vi "General_Test.vi"(8 "error in":errorcluster, 11 "Daten":T2={"Report.lvclass"=refnum, "Norm"="", "last State"=enum."Initialize", "Norm ID"=0, "parameter"=[], "EMTestCWS500N.lvclass"=refnum, "CEG4500.lvclass"=refnum, "Tektronix RSA5106A.lvclass"=refnum, "erfolgreich"=FALSE, "log"="", "Kommentar"="", "Device Enum"=enum."emTestCWS500N", "Test Enum"=enum."HF-Felder", "debug"=FALSE}) -> (0 "error out":errorcluster, 1 "Log":string, 2 "Daten out":T2={"Report.lvclass"=refnum, "Norm"="", "last State"=enum."Initialize", "Norm ID"=0, "parameter"=[], "EMTestCWS500N.lvclass"=refnum, "CEG4500.lvclass"=refnum, "Tektronix RSA5106A.lvclass"=refnum, "erfolgreich"=FALSE, "log"="", "Kommentar"="", "Device Enum"=enum."emTestCWS500N", "Test Enum"=enum."HF-Felder", "debug"=FALSE})   [LabVIEW 2013, in "EMV-Test.lvlib"]
uses:
  lib/EMV-Test.lvlib
  classes/Tests/TestInterface/Tests.ctl
  classes/Devices/DeviceInterface/Devices.ctl
  Main/controls/Data.ctl
  classes/Datastructure/Report/Report.lvclass
  classes/Devices/emTestCWS500N/EMTestCWS500N.lvclass
  classes/Devices/CEG4500/CEG4500.lvclass
  classes/Devices/Tektronix RSA5106A/Tektronix RSA5106A.lvclass
  Main/controls/State.ctl
  Main/controls/generalTestStates.ctl
  Main/controls/TestData.ctl
  Main/controls/TestStates.ctl
  lib/button_states.ctl
  classes/Devices/DeviceInterface/DeviceInterface.lvclass
  classes/Tests/TestInterface/TestInterface.lvclass
panel:
  in  "save Test":bool
  out "Status":T1
  in  "Custom Button 2":bool
  in  "Custom Button 1":bool
  in  "Button Referenzen":refnum<vi>[](array[refnum])
  in  "Neustart":bool
  out "device":T4=enum."Tektronix RSA5106A"
  out "test":T5=enum."Störaussendung"
  out "Parameter table":string[][](table) caption="Parameter"
  out "VISA resource name":refnum<visa-resource-name>="COM5"
  in  "Kommentar":string
  in  "Pause":bool
  in  "aktueller Test":string
  in  "manuell":bool
  in  "test laden":bool
  in  "Start":bool
  in  "Beenden":bool
  out "start":dbl format="%_19f"
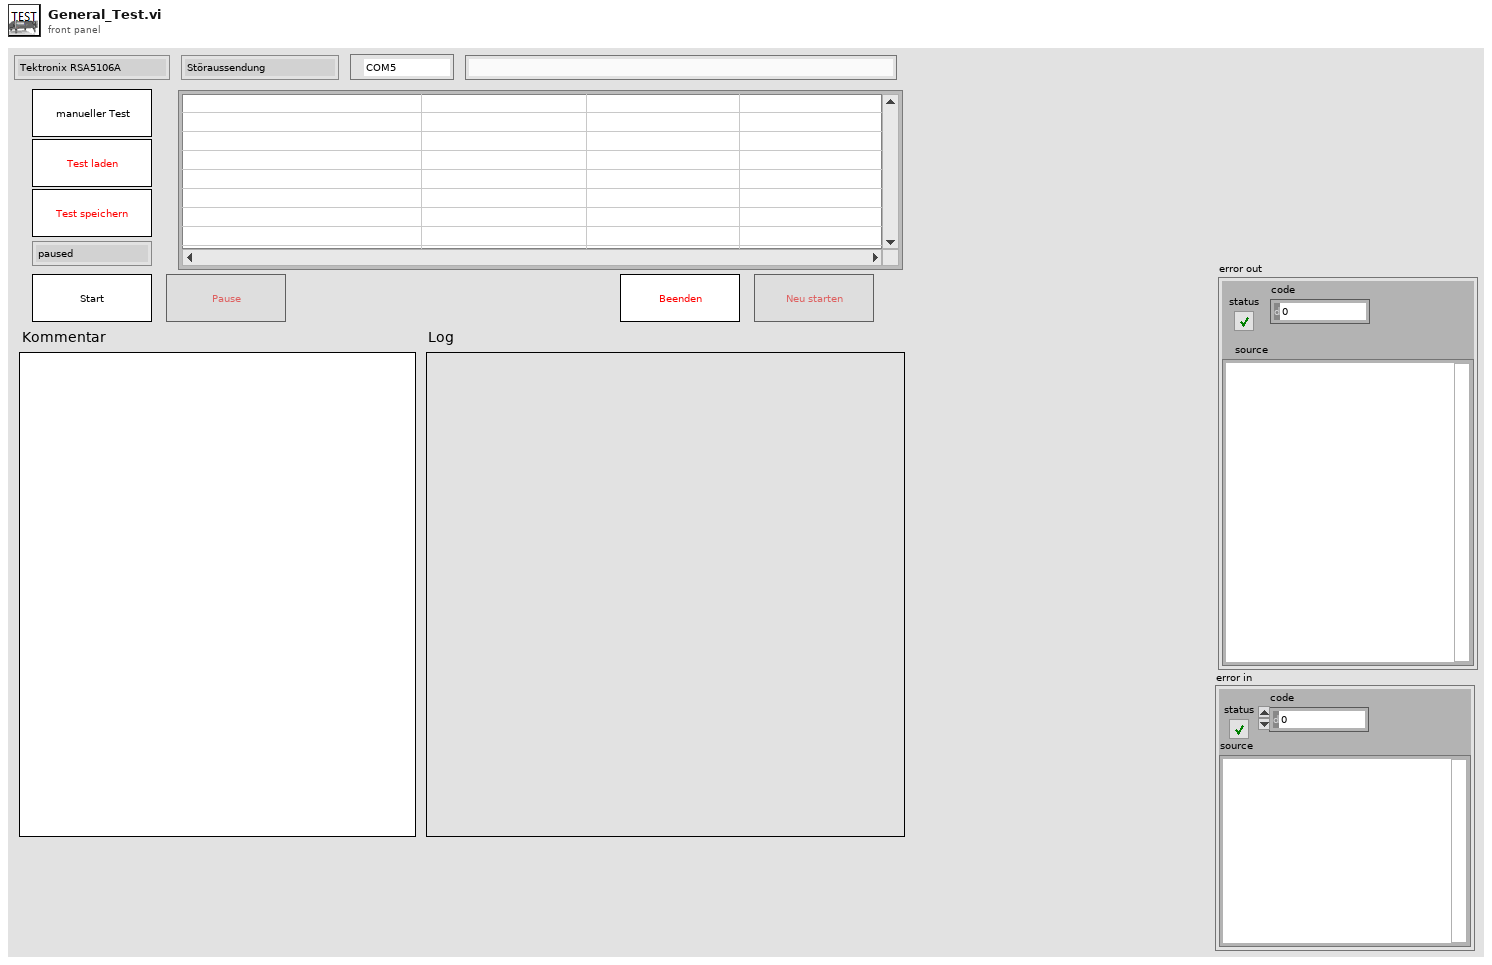
[diagram p1: front panel]
types:
  T1 = typedef "generalTestStates.ctl" = enum16{"paused", "starting", "waiting", "running", "finished"}
  T2 = typedef "Data.ctl" = cluster{"Report.lvclass":refnum<class "Report.lvclass">, "Norm":string, "last State":T3, "Norm ID":i32, "parameter":string[][], "EMTestCWS500N.lvclass":refnum<class "EMTestCWS500N.lvclass">, "CEG4500.lvclass":refnum<class "CEG4500.lvclass">, "Tektronix RSA5106A.lvclass":refnum<class "Tektronix RSA5106A.lvclass">, "erfolgreich":bool, "log":string, "Kommentar":string, "Device Enum":T4, "Test Enum":T5, "debug":bool}
  T3 = typedef "State.ctl" = enum16{"create Pdf", "load Report", "save Report", "do Test", "CDN Kalibrierung", "enter Report Parameters", "new Test", "Protokoll", "read Tree", "update Tree", "Fehler", "Initialize", "Wait for Event", "Exit"}
  T4 = typedef "Devices.ctl" = enum16{"unbekannt", "Tektronix RSA5106A", "emTestCWS500N", "CEG-4500"}
  T5 = typedef "Tests.ctl" = enum16{"unbekannt", "Störaussendung", "Burst", "ESD", "Surge", "Spannungseinbruch", "HF-Felder"}
  T6 = typedef "EMV-Test.lvlib/button_states.ctl" = enum16{"ende", "computing", "pause", "running", "start"}
  T7 = typedef "EMV-Test.lvlib/TestStates.ctl" = enum16{"event loop", "save Test", "Custom Action 1", "Custom Action 2", "pause", "vorgefertigter Test", "manueller Test", "respond to response", "error", "init", "start Test", "evaluate line", "wait for Response", "wait", "catch error", "close Connection", "end"}
  T8 = typedef "EMV-Test.lvlib/TestData.ctl" = cluster{"commandlist":string, "line":i32, "last response":string, "timeout":i32, "wait":u32, "erfolgreich":bool, "next state":T7, "Zustand":T1, "manual Test":bool}
  T9 = enum16{"open", "replace", "create", "open or create", "replace or create", "replace or create with confirmation"}
  T10 = enum16{"Left Button", "Center Button", "Right Button", "Window Close"}
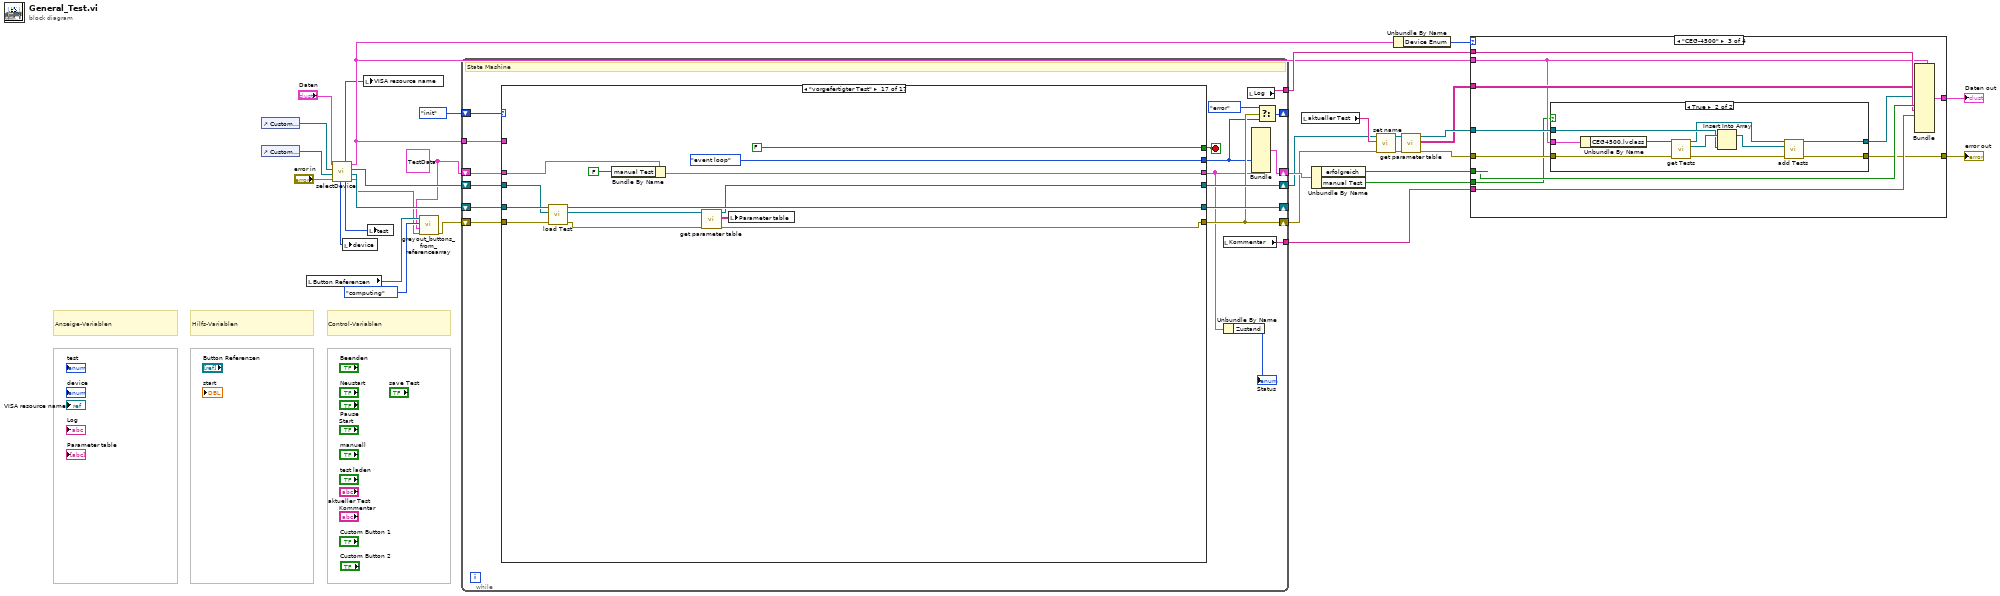
[diagram p0: block diagram]
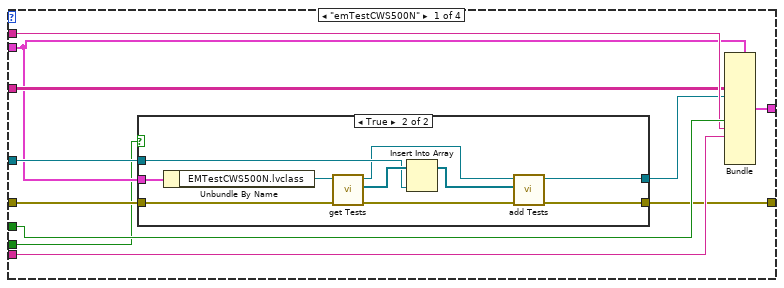
[diagram p2: hidden frame]
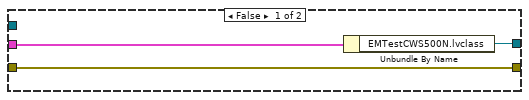
[diagram p3: hidden frame]
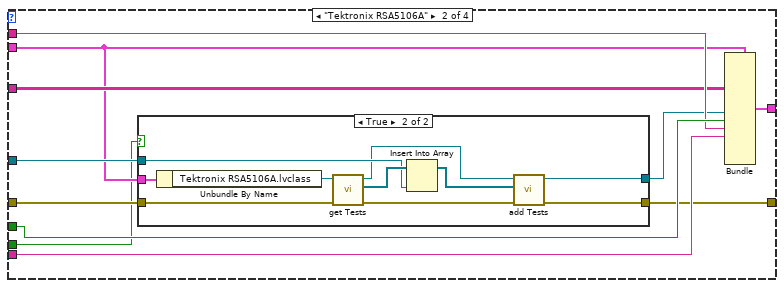
[diagram p4: hidden frame]
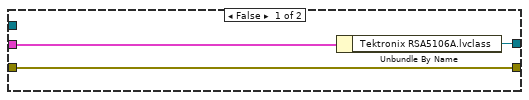
[diagram p5: hidden frame]
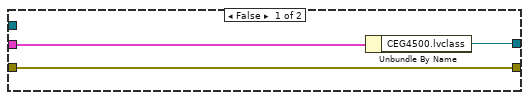
[diagram p6: hidden frame]
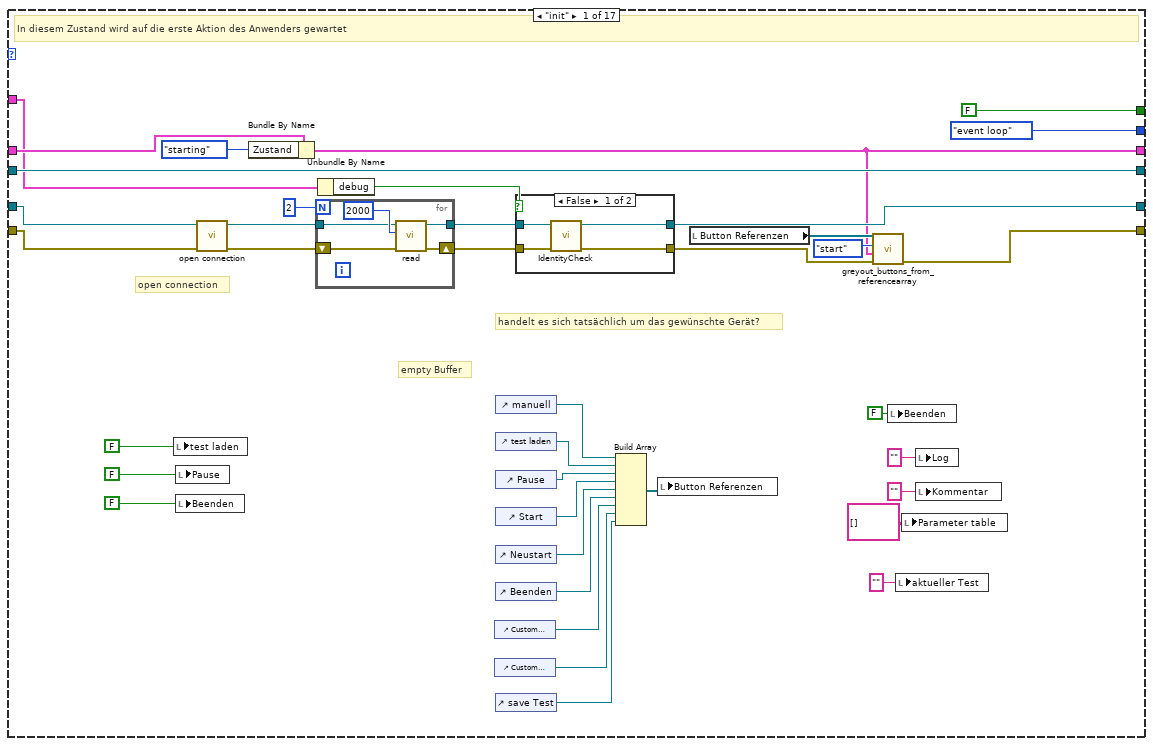
[diagram p8: hidden frame]
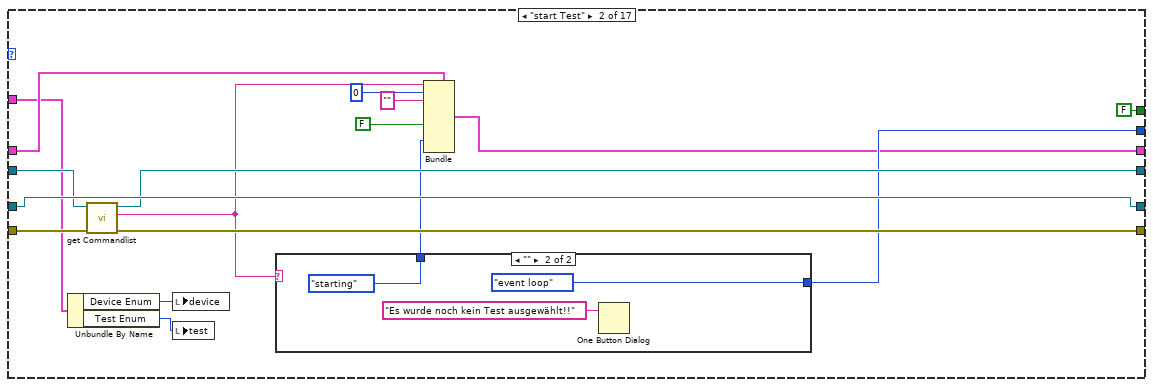
[diagram p10: hidden frame]
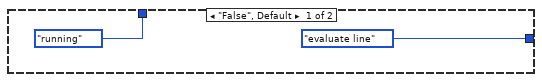
[diagram p11: hidden frame]
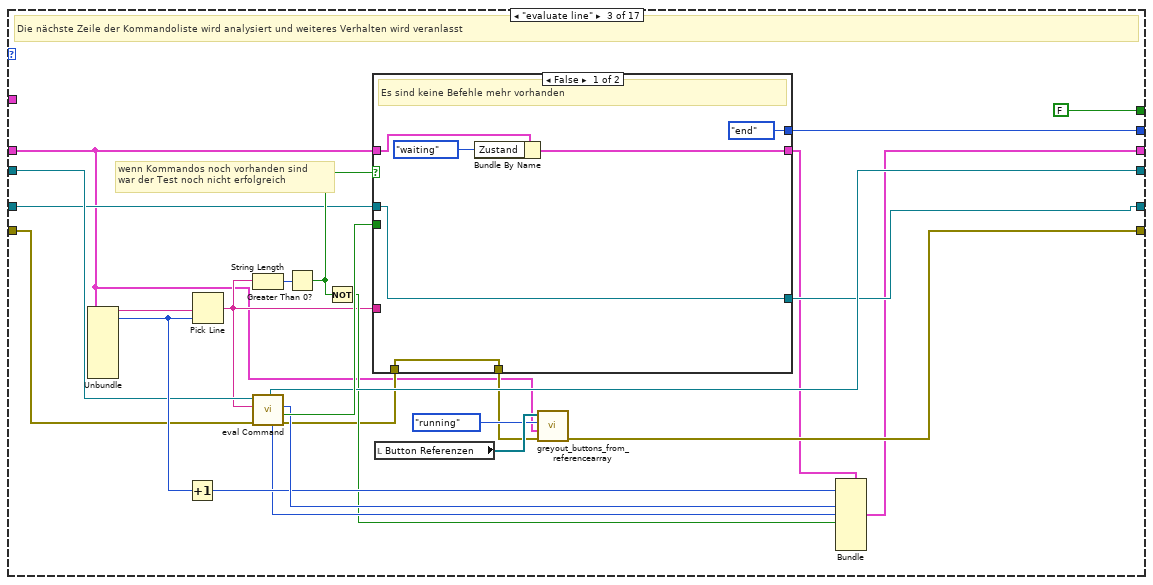
[diagram p12: hidden frame]
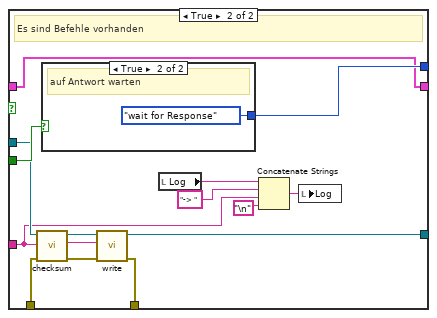
[diagram p13: hidden frame]
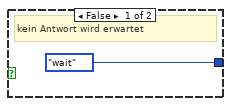
[diagram p14: hidden frame]
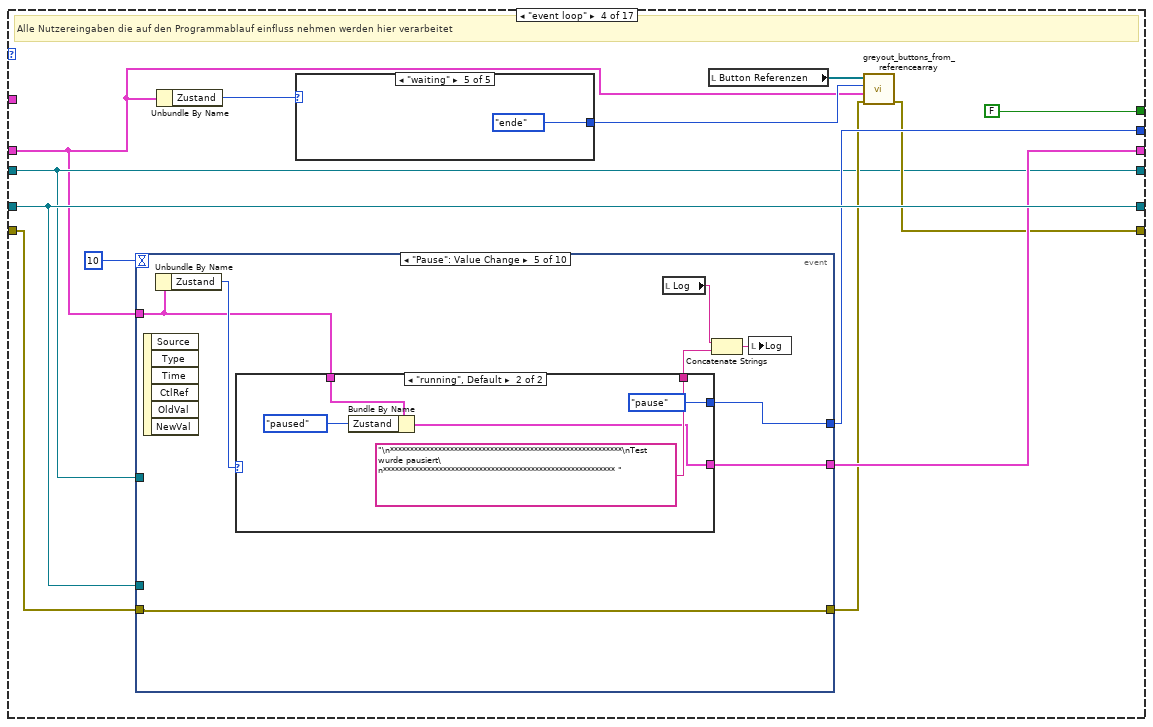
[diagram p15: hidden frame]
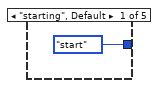
[diagram p16: hidden frame]
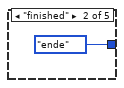
[diagram p17: hidden frame]
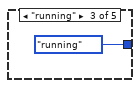
[diagram p18: hidden frame]
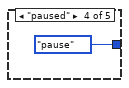
[diagram p19: hidden frame]
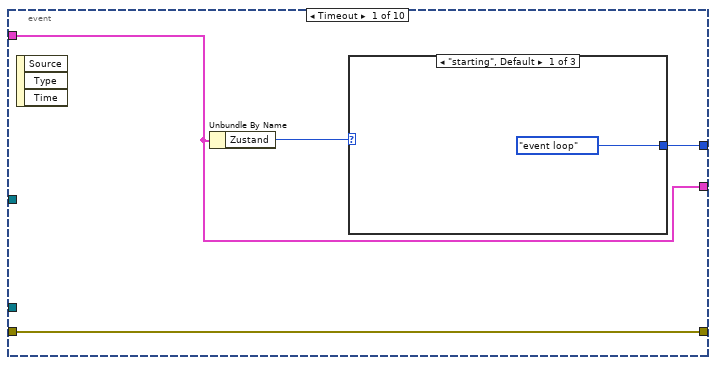
[diagram p20: hidden frame]
diagram:
  w3 = T8 {"commandlist"="", "line"=0, "last response"="", "timeout"=0, "wait"=0, "erfolgreich"=FALSE, "next state"=enum."event loop", "Zustand"=enum."starting", "manual Test"=FALSE}
  # "Hilfs-Variablen"
  # "Anzeige-Variablen"
  # "Control-Variablen"
  n1 = control-ref of="Custom Button 2"() -> (w24:refnum<vi>)
  n2 = control-ref of="Custom Button 1"() -> (w23:refnum<vi>)
  n3 = local read "Button Referenzen"() -> (w4:refnum<vi>[])
  n4 = call "selectDevice.vi"("error in (no error)"="error in", "Custom Button 1"=w23, "Custom Button 2"=w24, "Daten in"="Daten") -> ("error out"=w2:errorcluster, "DeviceInterface out"=w21:refnum<class "DeviceInterface.lvclass">, "Burst.lvclass"=w20:refnum<class "TestInterface.lvclass">, "Daten out"=w17:T2, "Test Enum"=w7:T5, "VISA resource name"=w6:refnum<visa-resource-name>, "Device Enum"=w8:T4)  [unwired: 1 in]
  n5 = local write "device"(w8) -> ()
  n6 = local write "VISA resource name"(w6) -> ()
  n7 = local write "test"(w7) -> ()
  n8 = call "greyout_buttons_from_referencearray.vi"("error in (no error)"=w2, 9:w3, "Enum"=button_states."computing", "Array"=w4) -> ("error out"=w1:errorcluster)  [unwired: 7 in]
  n9 = while {
    shift-right: [w41] -> _
    shift-left: TestStates."init" ("Enum") -> [w46]
    shift-right: [w39] -> w25
    shift-left: w1 -> [w44]
    shift-right: [w37] -> w32
    shift-left: w3 -> [w50]
    shift-right: [w43] -> _
    shift-left: w21 -> [w48]
    shift-right: [w47] -> w26
    shift-left: w20 -> [w45]
    tunnel: [w42] -> w29
    tunnel: [w36] -> w28
    tunnel: w17 -> [w33]
    stop <- w49 stop-if-true
    # "State Mashine"
    n10 = case shown="\"vorgefertigter Test\"" w46 {
      tunnel: w44 -> [w76 w111 w136 w179 w278 w310 w367 w390 w398 _ w441 w460 w469 w514 w537 w548 w565]
      tunnel: [w83 w108 w131 w174 w280 w320 w354 w390 w402 errorcluster {"status"=FALSE, "code"=0, "source"=""} ("error out") w424 w463 errorcluster {"status"=FALSE, "code"=0, "source"=""} ("error out") w507 w521 w548 w556] -> w39
      tunnel: [TestStates."event loop" ("Enum") w106 w125 w178 w272 w313 TestStates."catch error" ("Enum") TestStates."event loop" ("Enum") w401 TestStates."end" ("Enum") TestStates."event loop" ("Enum") w458 w474 w506 TestStates."event loop" ("Enum") TestStates."event loop" ("Enum") TestStates."event loop" ("Enum")] -> w38
      tunnel: w50 -> [w79 w115 w122 w170 w273 w315 w362 w388 w400 w415 w455 w457 w473 w508 w529 w551 w560]
      tunnel: [w66 w105 w123 w177 w274 w317 w363 w388 w400 w415 w455 w457 w472 w505 w527 w551 w558] -> w35
      tunnel: [FALSE FALSE FALSE FALSE FALSE FALSE FALSE FALSE FALSE TRUE FALSE FALSE FALSE FALSE FALSE FALSE FALSE] -> w49
      tunnel: w48 -> [w77 w112 w129 w180 w279 w316 w356 w392 w399 w419 w456 w464 w485 w511 w538 w549 w566]
      tunnel: w45 -> [w86 w110 w137 w171 w276 w311 w360 w393 w404 w420 w423 w461 w470 w513 w533 w550 w562]
      tunnel: [w86 w109 w141 w171 w275 w318 w360 w393 w404 w420 w423 w461 w470 w510 w523 w550 w555] -> w47
      tunnel: [w87 w112 w128 w180 w277 w319 w356 w392 w403 w419 w456 w464 w485 w511 w538 w549 w563] -> w43
      tunnel: w33 -> [w70 w100 _ _ w270 w307 _ _ _ w414 _ _ _ _ _ _ _]
      frame "init" {
        # "open connection"
        # "empty Buffer"
        # "handelt es sich tatsächlich um das gewünschte Gerät?"
        # "In diesem Zustand wird auf die erste Aktion des Anwenders gewartet"
        n11 = local write "test laden"(FALSE ("Beenden")) -> ()
        n12 = local write "Pause"(FALSE ("Beenden")) -> ()
        n13 = local write "Beenden"(FALSE ("Beenden")) -> ()
        n14 = call-dynamic "open connection.vi"("error in (no error)"=w76, "DeviceInterface Eingang"=w77) -> ("error out"=w73:errorcluster, "DeviceInterface Ausgang"=w74:refnum<class "DeviceInterface.lvclass">)  [unwired: 8 in]
        n15 = Bundle By Name(cluster=w79, "Zustand"=generalTestStates."starting") -> (w66:T8)
        n16 = for {
          N: 2 -> [_]
          tunnel: w74 -> [w90]
          shift-right: [w92] -> w71
          shift-left: w73 -> [w93]
          tunnel: [w89] -> w72
          n17 = call-dynamic "read.vi"("error in (no error)"=w93, "timeout (ms)"=2000, "DeviceInterface in"=w90) -> ("error out"=w92:errorcluster, "DeviceInterface out"=w89:refnum<class "DeviceInterface.lvclass">)  [unwired: 6 in, 1 out]
        }
        n18 = Unbundle By Name(w70) -> ("debug"=w85:bool)
        n19 = control-ref of="Custom Button 1"() -> (w62:refnum<vi>)
        n20 = control-ref of="Custom Button 2"() -> (w63:refnum<vi>)
        n21 = control-ref of="manuell"() -> (w59:refnum<vi>)
        n22 = control-ref of="test laden"() -> (w58:refnum<vi>)
        n23 = control-ref of="Pause"() -> (w57:refnum<vi>)
        n24 = control-ref of="Start"() -> (w56:refnum<vi>)
        n25 = control-ref of="Neustart"() -> (w55:refnum<vi>)
        n26 = control-ref of="Beenden"() -> (w61:refnum<vi>)
        n27 = control-ref of="save Test"() -> (w51:refnum<vi>)
        n28 = case shown="False" w85 {
          tunnel: w72 -> [w97 w99]
          tunnel: [w96 w99] -> w87
          tunnel: [w95 w98] -> w84
          tunnel: w71 -> [w94 w98]
          frame False {
            n29 = call-dynamic "IdentityCheck.vi"("error in (no error)"=w94, "DeviceInterface in"=w97) -> ("error out"=w95:errorcluster, "DeviceInterface out"=w96:refnum<class "DeviceInterface.lvclass">)  [unwired: 8 in]
          }
          frame True {
          }
        }
        n30 = Build Array(w59, w58, w57, w56, w55, w61, w62, w63, w51) -> (w60:refnum<vi>[])
        n31 = local write "Button Referenzen"(w60) -> ()
        n32 = local read "Button Referenzen"() -> (w82:refnum<vi>[])
        n33 = call "greyout_buttons_from_referencearray.vi"("error in (no error)"=w84, 9:w66, "Enum"=button_states."start", "Array"=w82) -> ("error out"=w83:errorcluster)  [unwired: 7 in]
        n34 = local write "Beenden"(FALSE ("Beenden")) -> ()
        n35 = local write "aktueller Test"("" ("Kommentar")) -> ()
        n36 = local write "Parameter table"(string[][] [] ("Parameter")) -> ()
        n37 = local write "Log"("" ("Log")) -> ()
        n38 = local write "Kommentar"("" ("Kommentar")) -> ()
      }
      frame "start Test" {
        n39 = Unbundle By Name(w100) -> ("Device Enum"=w101:T4, "Test Enum"=w102:T5)
        n40 = call-dynamic "get Commandlist.vi"("error in (no error)"=w111, "TestInterface (Eingang)"=w110) -> ("error out"=w108:errorcluster, "Commandlist"=w104:string, "TestInterface (Ausgang)"=w109:refnum<class "TestInterface.lvclass">)  [unwired: 7 in]
        n41 = local write "device"(w101) -> ()
        n42 = local write "test"(w102) -> ()
        n43 = case shown="\"\"" w104 {
          tunnel: [TestStates."evaluate line" ("Enum") TestStates."event loop" ("Enum")] -> w106
          tunnel: [generalTestStates."running" ("Zustand") generalTestStates."starting" ("Zustand")] -> w103
          frame "False", Default {
          }
          frame "" {
            n44 = One Button Dialog(message="Es wurde noch kein Test ausgewählt!!" ("Nachricht")) -> ()  [unwired: 1 in, 1 out]
          }
        }
        n45 = Bundle(cluster=w115, "commandlist"=w104, "line"=0, "last response"="", "erfolgreich"=FALSE, "Zustand"=w103) -> (w105:T8)  [unwired: 4 in]
      }
      frame "evaluate line" {
        # "wenn Kommandos noch vorhanden sind\nwar der Test noch nicht erfolgreich"
        # "Die nächste Zeile der Kommandoliste wird analysiert und weiteres Verhalten wird veranlasst"
        n46 = Unbundle(w122) -> ("commandlist"=w139:string, "line"=w144:i32)  [unwired: 7 out]
        n47 = Increment(x=w144) -> (x+1=w140:i32)
        n48 = Pick Line(multi-line string=w139, line index=w144) -> (output string=w130:string)  [unwired: 1 in]
        n49 = String Length(string=w130) -> (length=w146:i32)
        n50 = call "eval Command.vi"("error in (no error)"=w136, "Commandline"=w130, "TestInterface.lvclass"=w137) -> ("error out"=w127:errorcluster, "isQuerry"=w145:bool, "timeout(ms)"=w142:i32, "TestInterface.lvclass 2"=w141:refnum<class "TestInterface.lvclass">, "wait"=w138:u32)  [unwired: 4 in]
        n51 = Greater Than 0?(x=w146) -> (x > 0?=w134:bool)
        n52 = Not(x=w134) -> (.not. x?=w135:bool)
        n53 = case shown="False" w134 {
          tunnel: [TestStates."end" ("Enum") w166] -> w125
          tunnel: w145 -> [_ w167]
          tunnel: w130 -> [_ w154]
          tunnel: w129 -> [w150 w165]
          tunnel: w127 -> [w151 w164]
          tunnel: [w150 w160] -> w128
          tunnel: [w151 w159] -> w126
          tunnel: w122 -> [w149 w153]
          tunnel: [w147 w153] -> w124
          frame False {
            # "Es sind keine Befehle mehr vorhanden"
            n54 = Bundle By Name(cluster=w149, "Zustand"=generalTestStates."waiting") -> (w147:T8)
          }
          frame True {
            # "Es sind Befehle vorhanden"
            n55 = call-dynamic "checksum.vi"("error in (no error)"=w164, "input"=w154, "DeviceInterface in"=w165) -> ("error out"=w161:errorcluster, "output"=w162:string, "DeviceInterface out"=w163:refnum<class "DeviceInterface.lvclass">)  [unwired: 6 in]
            n56 = case shown="True" w167 {
              tunnel: [TestStates."wait" ("Enum") TestStates."wait for Response" ("Enum")] -> w166
              frame False {
                # "kein Antwort wird erwartet"
              }
              frame True {
                # "auf Antwort warten"
              }
            }
            n57 = call-dynamic "write.vi"("error in (no error)"=w161, "String to send"=w162, "DeviceInterface in"=w163) -> ("error out"=w159:errorcluster, "DeviceInterface out"=w160:refnum<class "DeviceInterface.lvclass">)  [unwired: 7 in]
            n58 = local read "Log"() -> (w158:string)
            n59 = Concatenate Strings(w158, "-> " ("string"), w154, "\n") -> (w156:string)
            n60 = local write "Log"(w156) -> ()
          }
        }
        n61 = local read "Button Referenzen"() -> (w133:refnum<vi>[])
        n62 = call "greyout_buttons_from_referencearray.vi"("error in (no error)"=w126, 9:w122, "Enum"=button_states."running", "Array"=w133) -> ("error out"=w131:errorcluster)  [unwired: 7 in]
        n63 = Bundle(cluster=w124, "line"=w140, "timeout"=w142, "wait"=w138, "erfolgreich"=w135) -> (w123:T8)  [unwired: 5 in]
      }
      frame "event loop" {
        # "Alle Nutzereingaben die auf den Programmablauf einfluss nehmen werden hier verarbeitet"
        n64 = event shown="[4] \"Pause\": Value Change" {
          selector: _ -> [_ _ _ _ _ _ _ _ _ _]
          dyn-events: _ -> [_ _ _ _ _ _ _ _ _ _]
          timeout: 10 -> [_ _ _ _ _ _ _ _ _ _]
          tunnel: [w190 w198 w199 w210 w218 w234 w246 w259 w265 w268] -> w175
          tunnel: w179 -> [w190 w198 w209 w210 w218 w234 w247 w259 w265 w268]
          tunnel: w180 -> [_ _ w208 _ _ _ _ _ _ _]
          tunnel: [w191 TestStates."manueller Test" ("Enum") TestStates."init" ("Enum") TestStates."save Test" ("Enum") w213 TestStates."end" ("Enum") TestStates."start Test" ("Enum") TestStates."vorgefertigter Test" ("Enum") TestStates."Custom Action 1" ("Enum") TestStates."Custom Action 2" ("Enum")] -> w178
          tunnel: w170 -> [w188 w196 w202 w211 w215 w233 w249 w260 w263 w267]
          tunnel: [w188 w196 w200 w211 w214 w231 w249 w260 w263 w267] -> w177
          tunnel: w171 -> [_ _ _ _ _ _ w245 _ _ _]
          event Timeout {
            n65 = event-data() -> ()  [unwired: 1 in, 3 out]
            n66 = Unbundle By Name(w188) -> ("Zustand"=w189:T1)
            n67 = case shown="\"starting\", Default" w189 {
              tunnel: [TestStates."event loop" ("Enum") TestStates."pause" ("Enum") TestStates."evaluate line" ("Enum")] -> w191
              frame "starting", Default {
              }
              frame "paused" {
              }
              frame "running" {
              }
            }
          }
          event "manuell": Value Change {
            n68 = event-data() -> ()  [unwired: 1 in, 6 out]
            n69 = local write "manuell"(FALSE ("manuell")) -> ()
          }
          event "Neustart": Value Change {
            n70 = event-data() -> ()  [unwired: 1 in, 6 out]
            n71 = call-dynamic "close connection.vi"("error in (no error)"=w209, "DeviceInterface in"=w208) -> ("error out"=w199:errorcluster)  [unwired: 8 in, 1 out]
            n72 = Bundle By Name(cluster=w202, "Zustand"=generalTestStates."starting") -> (w200:T8)
            n73 = local write "Neustart"(FALSE ("Neustart")) -> ()
            n74 = local read "Log"() -> (w205:string)
            n75 = Concatenate Strings(w205, "\n**********************************************************\nTest wurde neugestartet\n********************************************************** " ("string")) -> (w204:string)
            n76 = local write "Log"(w204) -> ()
          }
          event "save Test": Value Change {
            n77 = event-data() -> ()  [unwired: 1 in, 6 out]
          }
          event "Pause": Value Change {
            n78 = event-data() -> ()  [unwired: 1 in, 6 out]
            n79 = Unbundle By Name(w215) -> ("Zustand"=w216:T1)
            n80 = case shown="\"running\", Default" w216 {
              tunnel: ["\n**********************************************************\nTest wurde wiederaufgenommen\n********************************************************** " ("string") "\n**********************************************************\nTest wurde pausiert\n********************************************************** " ("string")] -> w217
              tunnel: w215 -> [w224 w229]
              tunnel: [w222 w227] -> w214
              tunnel: [TestStates."event loop" ("Enum") TestStates."pause" ("Enum")] -> w213
              frame "paused" {
                n81 = Bundle By Name(cluster=w224, "Zustand"=generalTestStates."running") -> (w222:T8)
              }
              frame "running", Default {
                n82 = Bundle By Name(cluster=w229, "Zustand"=generalTestStates."paused") -> (w227:T8)
              }
            }
            n83 = local read "Log"() -> (w220:string)
            n84 = Concatenate Strings(w220, w217) -> (w219:string)
            n85 = local write "Log"(w219) -> ()
          }
          event "Beenden": Value Change {
            n86 = event-data() -> ()  [unwired: 1 in, 6 out]
            n87 = Unbundle By Name(w233) -> ("erfolgreich"=w235:bool)
            n88 = case shown="False" w235 {
              tunnel: ["\n**********************************************************\nTest wurde erfolgreich beendet\n**********************************************************" ("string") "\n**********************************************************\nTest wurde durch den Anwender beendet\n**********************************************************" ("string")] -> w237
              frame True {
              }
              frame False {
              }
            }
            n89 = Bundle By Name(cluster=w233, "Zustand"=generalTestStates."finished") -> (w231:T8)
            n90 = local read "Log"() -> (w239:string)
            n91 = Concatenate Strings(w239, w237) -> (w238:string)
            n92 = local write "Log"(w238) -> ()
          }
          event "Start": Value Change {
            w243 = "\"" ("string")
            n93 = event-data() -> ()  [unwired: 1 in, 6 out]
            n94 = call-dynamic "get name.vi"("error in (no error)"=w247, "TestInterface (Eingang)"=w245) -> ("error out"=w246:errorcluster, "name"=w244:string)  [unwired: 7 in, 1 out]
            n95 = local write "Start"(FALSE ("Start")) -> ()
            n96 = local read "Log"() -> (w255:string)
            n97 = Get Date/Time String(want seconds? (F)=TRUE) -> (date string=w251:string, time string=w250:string)  [unwired: 2 out]
            n98 = call <vilib>:"Space Constant.vi"() -> ("String"=w252:string)
            n99 = Concatenate Strings(w255, "\n**********************************************************\nTest gestartet " ("string"), w251, w252, w250, w243, w244, w243, "\n**********************************************************\n\n" ("string")) -> (w256:string)
            n100 = local write "Log"(w256) -> ()
          }
          event "test laden": Value Change {
            n101 = event-data() -> ()  [unwired: 1 in, 6 out]
            n102 = local write "test laden"(FALSE ("standard")) -> ()
          }
          event "Custom Button 1": Value Change {
            n103 = event-data() -> ()  [unwired: 1 in, 6 out]
            n104 = local write "Custom Button 1"(FALSE ("Custom Button 1")) -> ()
          }
          event "Custom Button 2": Value Change {
            n105 = event-data() -> ()  [unwired: 1 in, 6 out]
            n106 = local write "Custom Button 2"(FALSE ("Custom Button 2")) -> ()
          }
        }
        n107 = Unbundle By Name(w170) -> ("Zustand"=w172:T1)
        n108 = case shown="\"waiting\"" w172 {
          tunnel: [button_states."start" ("Enum") button_states."ende" ("Enum") button_states."running" ("Enum") button_states."pause" ("Enum") button_states."ende" ("Enum")] -> w173
          frame "starting", Default {
          }
          frame "finished" {
          }
          frame "running" {
          }
          frame "paused" {
          }
          frame "waiting" {
          }
        }
        n109 = local read "Button Referenzen"() -> (w176:refnum<vi>[])
        n110 = call "greyout_buttons_from_referencearray.vi"("error in (no error)"=w175, 9:w170, "Enum"=w173, "Array"=w176) -> ("error out"=w174:errorcluster)  [unwired: 7 in]
      }
      frame "Custom Action 1" {
        # "eine Aktion die für ein Gerät speziell definiert werden kann"
        n111 = Unbundle By Name(w270) -> ("Device Enum"=w281:T4)
        n112 = case shown="\"Tektronix RSA5106A\"" w281 {
          tunnel: [w286 w306] -> w280
          tunnel: w279 -> [w285 w295]
          tunnel: w278 -> [w286 w289]
          tunnel: [w285 w294] -> w277
          tunnel: w276 -> [w284 w292]
          tunnel: [w284 w292] -> w275
          tunnel: [w283 w287] -> w274
          tunnel: w273 -> [w283 w287]
          tunnel: [TestStates."event loop" ("Enum") TestStates."event loop" ("Enum")] -> w272
          frame "unbekannt", Default {
          }
          frame "Tektronix RSA5106A" {
            n113 = local read "Button Referenzen"() -> (w291:refnum<vi>[])
            n114 = call "greyout_buttons_from_referencearray.vi"("error in (no error)"=w289, 9:w287, "Enum"=button_states."computing", "Array"=w291) -> ("error out"=w288:errorcluster)  [unwired: 7 in]
            n115 = Get Date/Time In Seconds() -> (seconds since 1Jan1904=w305:timestamp)
            n116 = Format Date/Time String(time format string (%c)="%d-%m-%Y-%H-%M-%S", seconds (now)=w305) -> (date/time string=w303:string)  [unwired: 1 in]
            n117 = Concatenate Strings("MMEMory:STORe:SCReen \"C:\\Users\\Spearfish\\Desktop\\Images\\Screencapture_" ("Command (Empty String)"), w303, "\"" ("string")) -> (w298:string)
            n118 = call-dynamic "write.vi"("error in (no error)"=w288, "String to send"=w298, "DeviceInterface in"=w295) -> ("error out"=w306:errorcluster, "DeviceInterface out"=w294:refnum<class "DeviceInterface.lvclass">)  [unwired: 7 in]
            n119 = local read "Log"() -> (w302:string)
            n120 = Concatenate Strings(w302, "-> " ("string"), w298, "\n") -> (w300:string)
            n121 = local write "Log"(w300) -> ()
          }
        }
      }
      frame "Custom Action 2" {
        # "eine Aktion die für ein Gerät speziell definiert werden kann"
        n122 = Unbundle By Name(w307) -> ("Device Enum"=w314:T4)
        n123 = call-dynamic "get name.vi"("error in (no error)"=w310, "TestInterface (Eingang)"=w311) -> ("error out"=w309:errorcluster, "name"=w308:string)  [unwired: 7 in, 1 out]
        n124 = case shown="\"Tektronix RSA5106A\"" w314 {
          tunnel: [w325 w340] -> w320
          tunnel: w316 -> [w324 w345]
          tunnel: w309 -> [w325 w336]
          tunnel: [w324 w328] -> w319
          tunnel: w311 -> [w323 w333]
          tunnel: [w323 w341] -> w318
          tunnel: [w322 w342] -> w317
          tunnel: w315 -> [w322 w342]
          tunnel: [TestStates."event loop" ("Enum") TestStates."event loop" ("Enum")] -> w313
          tunnel: w308 -> [_ w335]
          frame "unbekannt", Default {
          }
          frame "Tektronix RSA5106A" {
            n125 = local read "Button Referenzen"() -> (w344:refnum<vi>[])
            n126 = call-dynamic "get parameter table.vi"("error in (no error)"=w336, "TestInterface in"=w333) -> ("error out"=w327:errorcluster, "parameter table"=w334:string[][], "TestInterface out"=w332:refnum<class "TestInterface.lvclass">)  [unwired: 7 in]
            n127 = call "greyout_buttons_from_referencearray.vi"("error in (no error)"=w327, 9:w342, "Enum"=button_states."computing", "Array"=w344) -> ("error out"=w326:errorcluster)  [unwired: 7 in]
            n128 = for {
              N: 2 -> [_]
              tunnel: w345 -> [w349]
              shift-right: [w351] -> w337
              shift-left: w326 -> [w352]
              tunnel: [w348] -> w331
              n129 = call-dynamic "read.vi"("error in (no error)"=w352, "timeout (ms)"=2000, "DeviceInterface in"=w349) -> ("error out"=w351:errorcluster, "DeviceInterface out"=w348:refnum<class "DeviceInterface.lvclass">)  [unwired: 6 in, 1 out]
            }
            n130 = local read "Log"() -> (w330:string)
            n131 = call "readSettings.vi"("name"=w335, "error in"=w337, "log"=w330, "parameter table"=w334, "DeviceInterface in"=w331) -> ("error out"=w339:errorcluster, "log out"=w329:string, "parameter table out"=w338:string[][], "DeviceInterface out"=w328:refnum<class "DeviceInterface.lvclass">)  [unwired: 3 in]
            n132 = local write "Log"(w329) -> ()
            n133 = local write "Parameter table"(w338) -> ()
            n134 = call-dynamic "set parameter table.vi"("error in (no error)"=w339, "parameter table"=w338, "TestInterface in"=w332) -> ("error out"=w340:errorcluster, "TestInterface out"=w341:refnum<class "TestInterface.lvclass">)  [unwired: 7 in]
          }
        }
      }
      frame "wait for Response" {
        # "Die Antwort des Geräts wird erwartet, unter Umständen wird nach der Antwort noch eine Pause gemacht"
        n135 = Unbundle(w362) -> ("timeout"=w361:i32, "wait"=w357:u32)  [unwired: 7 out]
        n136 = flat-sequence {
          tunnel: w367 -> [w372]
          tunnel: [w372] -> w369
          tunnel: w356 -> [w371]
          tunnel: [w371] -> w355
          tunnel: [w377] -> w368
          tunnel: w369 -> [w376]
          tunnel: [w375] -> w366
          tunnel: w361 -> [w373]
          tunnel: w355 -> [w374]
          tunnel: w368 -> [w384]
          tunnel: w366 -> [w381]
          tunnel: [w384] -> w359
          tunnel: [w381] -> w358
          tunnel: [w385] -> w364
          tunnel: [w387] -> w354
          tunnel: w359 -> [w387]
          tunnel: w358 -> [w385]
          tunnel: w357 -> [w386]
          frame #0 {
            # "start timer"
            n137 = call <vilib>:"High Resolution Relative Seconds.vi"() -> ("relative seconds"=w370:dbl)
            n138 = local write "start"(w370) -> ()
          }
          frame #1 {
            # "read"
            n139 = call-dynamic "read.vi"("error in (no error)"=w376, "timeout (ms)"=w373, "DeviceInterface in"=w374) -> ("error out"=w377:errorcluster, "Return String"=w375:string)  [unwired: 6 in, 1 out]
          }
          frame #2 {
            # "write log"
            n140 = local read "start"() -> (w379:dbl)
            n141 = local read "Log"() -> (w383:string)
            n142 = call "TimerStop.vi"("Start Zeit"=w379) -> ("String"=w380:string)  [unwired: 10 in]
            n143 = Concatenate Strings(w383, w380, "<--" ("string"), w381) -> (w378:string)
            n144 = local write "Log"(w378) -> ()
          }
          frame #3 {
            # "wait"
            n145 = Wait (ms)(milliseconds to wait=w386) -> ()  [unwired: 1 out]
          }
        }
        n146 = Bundle(cluster=w362, "last response"=w364) -> (w363:T8)  [unwired: 8 in]
      }
      frame "wait" {
        # "Hier wird nur gewartet"
        n147 = Unbundle(w388) -> ("wait"=w391:u32)  [unwired: 8 out]
        n148 = Wait (ms)(milliseconds to wait=w391) -> ()  [unwired: 1 out]
      }
      frame "catch error" {
        n149 = call-dynamic "read.vi"("error in (no error)"=w398, "timeout (ms)"=2000, "DeviceInterface in"=w399) -> ("error out"=w397:errorcluster, "DeviceInterface out"=w396:refnum<class "DeviceInterface.lvclass">)  [unwired: 6 in, 1 out]
        n150 = call-dynamic "ErrorCatcher.vi"("error in (no error)"=w397, "Test Daten"=w400, "DeviceInterface in"=w396) -> ("error out"=w402:errorcluster, "DeviceInterface out"=w403:refnum<class "DeviceInterface.lvclass">)  [unwired: 7 in]
        n151 = case shown="Error" w402 {
          selector: w402 -> [_ w409]
          tunnel: [TestStates."respond to response" ("Enum") TestStates."error" ("Enum")] -> w401
          frame No Error {
          }
          frame Error {
            n152 = Unbundle(w409) -> ("source"=w408:string)  [unwired: 2 out]
            n153 = local read "Log"() -> (w412:string)
            n154 = Concatenate Strings(w412, "\n**********************************************************\nEin Fehler ist aufgetreten,Test wurde abgebrochen\nFehler:\n " ("string"), w408, "\n**********************************************************\n\n" ("string")) -> (w411:string)
            n155 = local write "Log"(w411) -> ()
          }
        }
      }
      frame "close Connection" {
        n156 = Unbundle By Name(w414) -> ("debug"=w417:bool)
        n157 = case shown="False" w417 {
          tunnel: w419 -> [w422 _]
          frame False {
            n158 = call-dynamic "close connection.vi"("DeviceInterface in"=w422) -> ()  [unwired: 9 in, 2 out]
          }
          frame True {
          }
        }
      }
      frame "save Test" {
        n159 = call <vilib>:"Get LV Class Name.vi"("error in (no error)"=w441, "object"=w423) -> ("class name"=w451:string)  [unwired: 8 in, 1 out]
        n160 = Match Pattern(string=w451, regular expression=".lvclass") -> (before substring=w452:string)  [unwired: 1 in, 3 out]
        n161 = Concatenate Strings(w452, "tests.json" ("string")) -> (w448:string)
        n162 = call <vilib>:"Application Directory.vi"() -> ("Application Directory"=w449:path)
        n163 = Build Path(base path=w449, name or relative path=w448) -> (appended path=w426:path)
        n164 = Open/Create/Replace File(file path (use dialog)=w426, operation (0:open)=T9."open or create", access (0:read/write)=enum16{"read/write", "read-only", "write-only"}."read-only") -> (refnum out=w444:refnum<file>, error out=w443:errorcluster)  [unwired: 3 in, 1 out]
        n165 = Read from Text File(file (use dialog)=w444, error in=w443) -> (refnum out=w427:refnum<file>, text=w442:string, error out=w429:errorcluster)  [unwired: 2 in, 1 out]
        n166 = Close File(refnum=w427, error in=w429) -> (error out=w428:errorcluster)  [unwired: 1 out]
        n167 = call "jsonToTest.vi"("error in (no error)"=w428, "JSON string"=w442) -> ("error out"=w437:errorcluster, "Tests"=w440:refnum<class "TestInterface.lvclass">[])  [unwired: 8 in]
        n168 = Build Array(w423) -> (w439:refnum<class "TestInterface.lvclass">[])
        n169 = Insert Into Array(array=w440, new element=w439) -> (w438:refnum<class "TestInterface.lvclass">[])  [unwired: 1 in]
        n170 = call "TestsToJson.vi"("error in (no error)"=w437, "Test Array"=w438) -> ("error out"=w431:errorcluster, "JSON string"=w430:string)  [unwired: 8 in]
        n171 = Open/Create/Replace File(file path (use dialog)=w426, error in=w431, operation (0:open)=T9."replace or create", access (0:read/write)=enum16{"read/write", "read-only", "write-only"}."write-only") -> (refnum out=w425:refnum<file>, error out=w432:errorcluster)  [unwired: 2 in, 1 out]
        n172 = Write to Text File(file (use dialog)=w425, text=w430, error in=w432) -> (refnum out=w434:refnum<file>, error out=w433:errorcluster)  [unwired: 1 in, 1 out]
        n173 = Close File(refnum=w434, error in=w433) -> (error out=w424:errorcluster)  [unwired: 1 out]
      }
      frame "end" {
        n174 = local read "Button Referenzen"() -> (w466:refnum<vi>[])
        n175 = call "greyout_buttons_from_referencearray.vi"("error in (no error)"=w460, 9:w457, "Enum"=button_states."ende", "Array"=w466) -> ("error out"=w463:errorcluster)  [unwired: 7 in]
        n176 = Unbundle By Name(w457) -> ("Zustand"=w462:T1)
        n177 = case shown="\"waiting\", Default" w462 {
          tunnel: [TestStates."event loop" ("Enum") TestStates."close Connection" ("Enum")] -> w458
          frame "waiting", Default {
          }
          frame "finished" {
          }
        }
      }
      frame "error" {
        n178 = Unbundle(w469) -> ("source"=w482:string)  [unwired: 2 out]
        n179 = Concatenate Strings("Es ist ein Fehler aufgetreten:\n" ("String"), w482, "\nMöchten Sie den Test weiter führen ? Oder neu starten ?" ("String")) -> (w480:string)
        n180 = call <vilib>:"Three Button Dialog.vi"("Allow user to close window? (TRUE)"=FALSE, "Window Title (\"\")"="Fehlermeldung" ("Window Title (\"\")"), "Right Button Text (\"Cancel\")"="Abbrechen" ("Right Button Text (\"Cancel\")"), "Center Button Text (\"No\")"="Neu starten" ("Center Button Text (\"No\")"), "Left Button Text (\"Yes\")"="Weiter" ("Left Button Text (\"Yes\")"), "message"=w480) -> ("Which Button?"=w475:T10)  [unwired: 5 in]
        n181 = case shown="\"Left Button\", Default" w475 {
          tunnel: [w487 TestStates."close Connection" ("Enum") TestStates."init" ("Enum")] -> w474
          tunnel: w473 -> [w488 w497 w503]
          tunnel: [w488 w495 w500] -> w472
          tunnel: w469 -> [_ w489 _]
          frame "Left Button", Default {
            n182 = Unbundle By Name(w488) -> ("next state"=w487:T7)
          }
          frame "Right Button" {
            n183 = Unbundle By Name(w489) -> ("source"=w490:string)
            n184 = Bundle By Name(cluster=w497, "Zustand"=generalTestStates."finished") -> (w495:T8)
            n185 = local read "Log"() -> (w491:string)
            n186 = Concatenate Strings(w491, "\n**********************************************************\nDer Test wurde vorzeitig wegen eines Fehlers beendet\n " ("Log"), w490, "\n**********************************************************") -> (w492:string)
            n187 = local write "Log"(w492) -> ()
          }
          frame "Center Button" {
            n188 = Bundle By Name(cluster=w503, "line"=0, "erfolgreich"=FALSE, "Zustand"=generalTestStates."starting") -> (w500:T8)
          }
        }
      }
      frame "respond to response" {
        n189 = call-dynamic "respond to response.vi"("error in (no error)"=w514, 10:w508, "TestInterface Eingang"=w513) -> ("error out"=w507:errorcluster, "read again?"=w509:bool, "Cluster"=w505:T8, "TestInterface Ausgang"=w510:refnum<class "TestInterface.lvclass">)  [unwired: 5 in]
        n190 = case shown="No Error" w507 {
          tunnel: [w516 TestStates."error" ("Enum")] -> w506
          tunnel: w509 -> [w515 _]
          frame No Error {
            n191 = case shown="False" w515 {
              tunnel: [TestStates."event loop" ("Enum") TestStates."wait for Response" ("Enum")] -> w516
              frame False {
              }
              frame True {
                # "read again ?"
              }
            }
          }
          frame Error {
          }
        }
      }
      frame "manueller Test" {
        n192 = call-dynamic "manual test UI.vi"("error in (no error)"=w537, "TestInterface Eingang"=w533) -> ("error out"=w536:errorcluster, "abbrechen"=w520:bool, "Parameters"=w535:u32[], "TestInterface Ausgang"=w534:refnum<class "TestInterface.lvclass">)  [unwired: 6 in]
        n193 = case shown="False" w520 {
          tunnel: w534 -> [w541 _]
          tunnel: w536 -> [w540 w546]
          tunnel: [w542 w545] -> w532
          tunnel: [w543 w546] -> w530
          tunnel: w535 -> [w544 _]
          tunnel: w533 -> [_ w545]
          frame False {
            n194 = call-dynamic "CheckParameters.vi"("error in (no error)"=w540, "Parameters"=w544, "TestInterface in"=w541) -> ("error out"=w543:errorcluster, "TestInterface out"=w542:refnum<class "TestInterface.lvclass">)  [unwired: 7 in]
          }
          frame True {
          }
        }
        n195 = Not(x=w520) -> (.not. x?=w528:bool)
        n196 = Bundle By Name(cluster=w529, "manual Test"=w528) -> (w527:T8)
        n197 = call-dynamic "get name.vi"("error in (no error)"=w530, "TestInterface (Eingang)"=w532) -> ("error out"=w524:errorcluster, "name"=w531:string, "TestInterface (Ausgang)"=w525:refnum<class "TestInterface.lvclass">)  [unwired: 7 in]
        n198 = local write "aktueller Test"(w531) -> ()
        n199 = call-dynamic "get parameter table.vi"("error in (no error)"=w524, "TestInterface in"=w525) -> ("error out"=w521:errorcluster, "parameter table"=w522:string[][], "TestInterface out"=w523:refnum<class "TestInterface.lvclass">)  [unwired: 7 in]
        n200 = local write "Parameter table"(w522) -> ()
      }
      frame "pause" {
      }
      frame "vorgefertigter Test" {
        n201 = call-dynamic "load Test.vi"("error in (no error)"=w565, "irgendein Test"=w562, "DeviceInterface Eingang"=w566) -> ("error out"=w553:errorcluster, "TestInterface.lvclass"=w554:refnum<class "TestInterface.lvclass">, "DeviceInterface Ausgang"=w563:refnum<class "DeviceInterface.lvclass">)  [unwired: 6 in]
        n202 = Bundle By Name(cluster=w560, "manual Test"=FALSE) -> (w558:T8)
        n203 = call-dynamic "get parameter table.vi"("error in (no error)"=w553, "TestInterface in"=w554) -> ("error out"=w556:errorcluster, "parameter table"=w557:string[][], "TestInterface out"=w555:refnum<class "TestInterface.lvclass">)  [unwired: 7 in]
        n204 = local write "Parameter table"(w557) -> ()
      }
    }
    n205 = local read "Kommentar"() -> (w36:string)
    n206 = Unbundle By Name(w35) -> ("Zustand"=→"Status":T1)
    n207 = local read "Log"() -> (w42:string)
    n208 = Bundle(cluster=w35, "next state"=w38) -> (w37:T8)  [unwired: 8 in]
    n209 = Select(t=TestStates."error" ("Enum"), s=w39, f=w38) -> (s? t:f=w41:T7)
  }
  n210 = local read "aktueller Test"() -> (w27:string)
  n211 = Unbundle By Name(w32) -> ("erfolgreich"=w31:bool, "manual Test"=w15:bool)
  n212 = call-dynamic "set name.vi"("error in (no error)"=w25, "name"=w27, "TestInterface (Eingang)"=w26) -> ("error out"=w12:errorcluster, "TestInterface (Ausgang)"=w13:refnum<class "TestInterface.lvclass">)  [unwired: 7 in]
  n213 = Unbundle By Name(w17) -> ("Device Enum"=w19:T4)
  n214 = call-dynamic "get parameter table.vi"("error in (no error)"=w12, "TestInterface in"=w13) -> ("error out"=w9:errorcluster, "parameter table"=w10:string[][], "TestInterface out"=w11:refnum<class "TestInterface.lvclass">)  [unwired: 7 in]
  n215 = case shown="\"CEG-4500\"" w19 {
    tunnel: w31 -> [w577 w601 w625 _]
    tunnel: w29 -> [w576 w600 w624 _]
    tunnel: w28 -> [w575 w599 w623 _]
    tunnel: w11 -> [w574 w598 w622 _]
    tunnel: w9 -> [w573 w597 w621 w640]
    tunnel: [w572 w596 w620 w640] -> w30
    tunnel: [w569 w593 w619 w639] -> w18
    tunnel: w10 -> [w570 w595 w618 _]
    tunnel: w17 -> [w568 w592 w616 w639]
    tunnel: w15 -> [w567 w591 w615 _]
    frame "emTestCWS500N" {
      n216 = case shown="True" w567 {
        tunnel: w574 -> [_ w588]
        tunnel: w573 -> [w580 w584]
        tunnel: [w580 w583] -> w572
        tunnel: [w579 w582] -> w571
        tunnel: w568 -> [w578 w581]
        frame False {
          n217 = Unbundle By Name(w578) -> ("EMTestCWS500N.lvclass"=w579:refnum<class "EMTestCWS500N.lvclass">)
        }
        frame True {
          n218 = Unbundle By Name(w581) -> ("EMTestCWS500N.lvclass"=w590:refnum<class "EMTestCWS500N.lvclass">)
          n219 = call-dynamic "get Tests.vi"("error in (no error)"=w584, "DeviceInterface (Eingang)"=w590) -> ("error out"=w585:errorcluster, "Tests"=w589:refnum<class "TestInterface.lvclass">[], "DeviceInterface (Ausgang)"=w586:refnum<class "EMTestCWS500N.lvclass">)  [unwired: 7 in]
          n220 = Insert Into Array(array=w589, new element=w588) -> (w587:refnum<class "TestInterface.lvclass">[])  [unwired: 1 in]
          n221 = call-dynamic "add Tests.vi"("error in (no error)"=w585, "Tests"=w587, "DeviceInterface (Eingang)"=w586) -> ("error out"=w583:errorcluster, "DeviceInterface (Ausgang)"=w582:refnum<class "EMTestCWS500N.lvclass">)  [unwired: 7 in]
        }
      }
      n222 = Bundle(cluster=w568, "parameter"=w570, "EMTestCWS500N.lvclass"=w571, "erfolgreich"=w577, "log"=w576, "Kommentar"=w575) -> (w569:T2)  [unwired: 9 in]
    }
    frame "Tektronix RSA5106A" {
      n223 = case shown="True" w591 {
        tunnel: w598 -> [_ w612]
        tunnel: w597 -> [w604 w608]
        tunnel: [w604 w607] -> w596
        tunnel: [w603 w606] -> w594
        tunnel: w592 -> [w602 w605]
        frame False {
          n224 = Unbundle By Name(w602) -> ("Tektronix RSA5106A.lvclass"=w603:refnum<class "Tektronix RSA5106A.lvclass">)
        }
        frame True {
          n225 = Unbundle By Name(w605) -> ("Tektronix RSA5106A.lvclass"=w614:refnum<class "Tektronix RSA5106A.lvclass">)
          n226 = call-dynamic "get Tests.vi"("error in (no error)"=w608, "DeviceInterface (Eingang)"=w614) -> ("error out"=w609:errorcluster, "Tests"=w613:refnum<class "TestInterface.lvclass">[], "DeviceInterface (Ausgang)"=w610:refnum<class "Tektronix RSA5106A.lvclass">)  [unwired: 7 in]
          n227 = Insert Into Array(array=w613, new element=w612) -> (w611:refnum<class "TestInterface.lvclass">[])  [unwired: 1 in]
          n228 = call-dynamic "add Tests.vi"("error in (no error)"=w609, "Tests"=w611, "DeviceInterface (Eingang)"=w610) -> ("error out"=w607:errorcluster, "DeviceInterface (Ausgang)"=w606:refnum<class "Tektronix RSA5106A.lvclass">)  [unwired: 7 in]
        }
      }
      n229 = Bundle(cluster=w592, "parameter"=w595, "Tektronix RSA5106A.lvclass"=w594, "erfolgreich"=w601, "log"=w600, "Kommentar"=w599) -> (w593:T2)  [unwired: 9 in]
    }
    frame "CEG-4500" {
      n230 = case shown="True" w615 {
        tunnel: w622 -> [_ w636]
        tunnel: w621 -> [w627 w632]
        tunnel: [w627 w631] -> w620
        tunnel: [w628 w630] -> w617
        tunnel: w616 -> [w626 w629]
        frame False {
          n231 = Unbundle By Name(w626) -> ("CEG4500.lvclass"=w628:refnum<class "CEG4500.lvclass">)
        }
        frame True {
          n232 = Unbundle By Name(w629) -> ("CEG4500.lvclass"=w638:refnum<class "CEG4500.lvclass">)
          n233 = call-dynamic "get Tests.vi"("error in (no error)"=w632, "DeviceInterface (Eingang)"=w638) -> ("error out"=w633:errorcluster, "Tests"=w637:refnum<class "TestInterface.lvclass">[], "DeviceInterface (Ausgang)"=w634:refnum<class "CEG4500.lvclass">)  [unwired: 7 in]
          n234 = Insert Into Array(array=w637, new element=w636) -> (w635:refnum<class "TestInterface.lvclass">[])  [unwired: 1 in]
          n235 = call-dynamic "add Tests.vi"("error in (no error)"=w633, "Tests"=w635, "DeviceInterface (Eingang)"=w634) -> ("error out"=w631:errorcluster, "DeviceInterface (Ausgang)"=w630:refnum<class "CEG4500.lvclass">)  [unwired: 7 in]
        }
      }
      n236 = Bundle(cluster=w616, "parameter"=w618, "CEG4500.lvclass"=w617, "erfolgreich"=w625, "log"=w624, "Kommentar"=w623) -> (w619:T2)  [unwired: 9 in]
    }
    frame "unbekannt" {
    }
  }
  "error out" <- w30
  "Daten out" <- w18
